vi "PH_Timing.Action Switch Interlock Bypass.vi"(0 "i ref in":refnum<vi>, 5 "error in (no error)":errorcluster) -> (14 "i ref out":refnum<vi>, 19 "error out":errorcluster)   [LabVIEW 2014, in "PH_Timing.lvlib"]
doc: "Within this VI the action of the related event case is done: the timing interlock switch is switched."
uses:
  PH_Timing.lvlib
  PH_Basics/PH_PP_Common/PH_PP_Common.PUs.ctl
  PH_Classes/PH_Switch/PH_Switch.lvlib
  PH_Basics/PH_PP_Common/PH_PP_Common.lvlib
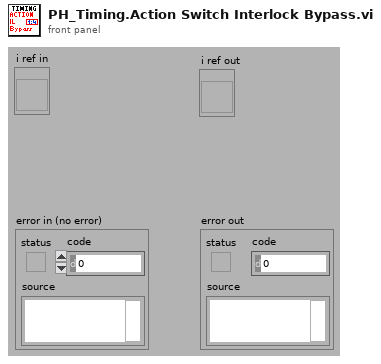
[diagram p1: front panel]
types:
  T1 = typedef "PH_PP_Common.lvlib/PH_PP_Common.PUs.ctl" = enum16{"no Info", "PA-19mm-1", "PA-19mm-2", "PA-45mm-PILC", "PA-45mm-MAIN", "MA-PU-1", "MA-PU-2", "MA-PU-3", "MA-PU-4", "MA-PU-5", "MA-PU-6", "MA-FR", "MA-PILC", "PA-45mm-DP"}
  T2 = typedef "PH_Timing.lvlib/PH_Timing.i attribute.ctl" = cluster{"Sequencer":cluster{"linked?":bool, "Proc State":string, "Ref State":refnum<vi>}, "Gate Generator":cluster{"GD":cluster{"Device Status":T3, "linked?":bool}, "Settings":T4, "GUI Ref":refnum<vi>}, "Interlock Bypass":cluster{"Instancename":string, "Switch linked?":bool, "Device Status":T3, "Ref Status":refnum<vi>}, "Roughtuner":cluster{"Settings":T5, "GUI Ref":refnum<vi>, "GD":cluster{"Device Status":T3, "linked?":bool}}, "0,5Hz Gater":cluster{"Settings":T6, "GUI Ref":refnum<vi>, "GD":cluster{"Device Status":T3, "linked?":bool}}, "Slow Trigger":cluster{"Settings":T7, "GUI Ref":refnum<vi>, "Service ID Delay":i32, "Service ID Ext Trig":i32, "Wanted Settings":T7}, "Timing Mode":cluster{"Mode":T8, "GUI Ref":refnum<vi>, "Service ID T2":i32, "Service ID Mode":i32, "Wanted Mode":T8}, "ns Generator":cluster{"Settings":T9, "ns Generator Settings":refnum<vi>, "GD":cluster{"Device Status":T3, "linked?":bool}}, "Phase FEs":cluster{"Settings":T12, "GUI Ref":refnum<vi>, "Service ID Phase":i32, "Wanted Settings":T12}, "GD GUI Refs":refnum<vi>[], "Heads":T13[], "GUI Ref Delete":refnum<vi>}
  T3 = typedef "PH_StatusHandler.lvlib/PH_StatusHandler.Status.ctl" = i16
  T4 = typedef "PH_Timing.lvlib/PH_Timing.GateGen.ctl" = cluster{"Instance":string, "Channel Gate":i32, "Channel T2":i32, "Width Gate":dbl, "Width T2":dbl, "Delay Gate":dbl, "Delay T2":dbl, "Gate activ":bool, "T2 activ":bool, "System Mode":enum16{"Normal", "Single", "Burst", "Duty Cycle"}}
  T5 = typedef "PH_Timing.lvlib/PH_Timing.Roughtuner.ctl" = cluster{"Instance":string, "Phase PHELIX / UNILAC":cluster{"Channel":u16, "relative to":u16, "Delay [ms]":dbl}, "Pulse Length":cluster{"Channel":u16, "relative to":u16, "Delay [ms]":dbl}, "Trigger":cluster{"externally?":bool, "Rate [Hz]":dbl}}
  T6 = typedef "PH_Timing.lvlib/PH_Timing.0.5HzGater.ctl" = cluster{"Instance":string, "Channel ns FE Delay":i32, "Channel 0.5Hz":i32, "Width ns FE Delay":dbl, "Width 0.5Hz":dbl, "Delay ns FE Delay":dbl, "Delay 0.5Hz":dbl, "ns FE Delay active":bool, "0.5Hz activ":bool, "ns FE Delay inverted":bool, "0.5Hz inverted":bool}
  T7 = typedef "PH_Timing.lvlib/PH_Timing.Slow Trigger Settings.ctl" = cluster{"Delay":dbl, "externally triggered?":bool}
  T8 = typedef "PH_Timing.lvlib/PH_Timing.Timing Mode.ctl" = cluster{"T2":i16, "Modeselector":enum32{"10 Hz", "0.5 Hz", "Shot"}}
  T9 = typedef "PH_Timing.lvlib/PH_Timing.ns Generator.ctl" = cluster{"Instance":string, "Phase fs / ns FE":cluster{"Channel":T10, "Settings":T11}}
  T10 = typedef "Stanford Research DG645 - Driver.lvlib/Channel.ctl" = i32
  T11 = typedef "PH_SRDG645.lvlib/PH_SRDG645.Channel Settings.ctl" = cluster{"Delay [s]":dbl, "relative to":i32}
  T12 = typedef "PH_Timing.lvlib/PH_Timing.Phase FEs.ctl" = cluster{"Phase":dbl}
  T13 = typedef "PH_Timing.lvlib/PH_Timing.PU Data.ctl" = cluster{"linked?":bool, "Data":T14, "GD":cluster{"Device Status":T3, "linked?":bool}, "GUI Ref":refnum<vi>, "PU":T1}
  T14 = typedef "PH_Timing.lvlib/PH_Timing.PU Info.ctl" = cluster{"Act CH?":bool, "GD":string, "CH":i32, "Delay":dbl, "active":bool, "in Use?":bool}
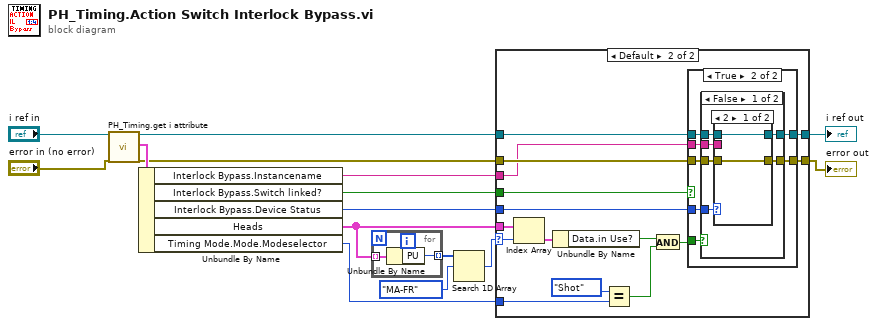
[diagram p0: block diagram]
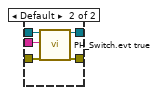
[diagram p4: hidden frame]
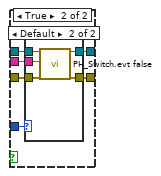
[diagram p5: hidden frame]
diagram:
  n1 = call "PH_Timing.get i attribute.vi"("i ref in"="i ref in", "error in (no error)"="error in (no error)") -> ("i ref out"=w10:refnum<vi>, "i attribute"=w11:T2, "error out"=w9:errorcluster)  [unwired: 15 in]
  n2 = Unbundle By Name(w11) -> ("Interlock Bypass.Instancename"=w8:string, "Interlock Bypass.Switch linked?"=w4:bool, "Interlock Bypass.Device Status"=w1:T3, "Heads"=w3:T13[], "Timing Mode.Mode.Modeselector"=w2:enum32{"10 Hz", "0.5 Hz", "Shot"})
  n3 = for {
    tunnel: w3 -> [w17] mode=indexing
    tunnel: [w16] -> w7 mode=indexing
    n4 = Unbundle By Name(w17) -> ("PU"=w16:T1)
  }
  n5 = Search 1D Array(1D array=w7, element=PH_PP_Common.PUs."MA-FR") -> (index of element=w5:i32)  [unwired: 1 in]
  n6 = case shown="Default" w5 {
    selector: w5 -> [_ w28]
    tunnel: [w19 w34] -> w13
    tunnel: [w18 w33] -> w12
    tunnel: w10 -> [w19 w32]
    tunnel: w9 -> [w18 w31]
    tunnel: w8 -> [_ w30]
    tunnel: w2 -> [_ w26]
    tunnel: w3 -> [_ w29]
    tunnel: w4 -> [_ w21]
    tunnel: w1 -> [_ w20]
    frame -1 {
    }
    frame Default {
      n7 = Index Array(array=w29, index=w28) -> (element=w27:T13)
      n8 = Unbundle By Name(w27) -> ("Data.in Use?"=w22:bool)
      n9 = Equal?(x=enum32{"10 Hz", "0.5 Hz", "Shot"}."Shot" ("y"), y=w26) -> (x = y?=w23:bool)
      n10 = And(x=w22, y=w23) -> (x .and. y?=w24:bool)
      n11 = case shown="True" w21 {
        tunnel: w32 -> [w36 w43]
        tunnel: [w36 w42] -> w34
        tunnel: w31 -> [w35 w41]
        tunnel: [w35 w40] -> w33
        tunnel: w30 -> [_ w39]
        tunnel: w24 -> [_ w38]
        tunnel: w20 -> [_ w37]
        frame False {
        }
        frame True {
          n12 = case shown="False" w38 {
            tunnel: [w49 w59] -> w42
            tunnel: [w48 w61] -> w40
            tunnel: w43 -> [w47 w60]
            tunnel: w41 -> [w46 w62]
            tunnel: w39 -> [w45 w58]
            tunnel: w37 -> [w44 w57]
            frame False {
              n13 = case shown="2" w44 {
                tunnel: [w51 w56] -> w49
                tunnel: [w50 w55] -> w48
                tunnel: w47 -> [w51 w54]
                tunnel: w46 -> [w50 w53]
                tunnel: w45 -> [_ w52]
                frame 2 {
                }
                frame Default {
                  n14 = call "PH_Switch.evt true.vi"("i ref in"=w54, "Instance"=w52, "error in (no error)"=w53) -> ("i ref out"=w56:refnum<vi>, "error out"=w55:errorcluster)  [unwired: 15 in]
                }
              }
            }
            frame True {
              n15 = case shown="Default" w57 {
                tunnel: w62 -> [w63 w69]
                tunnel: [w63 w68] -> w61
                tunnel: w60 -> [w64 w67]
                tunnel: [w64 w66] -> w59
                tunnel: w58 -> [_ w65]
                frame 1 {
                }
                frame Default {
                  n16 = call "PH_Switch.evt false.vi"("i ref in"=w67, "Instance"=w65, "error in (no error)"=w69) -> ("i ref out"=w66:refnum<vi>, "error out"=w68:errorcluster)  [unwired: 15 in]
                }
              }
            }
          }
        }
      }
    }
  }
  "error out" <- w12
  "i ref out" <- w13
